vi "OPEN EXCEL.vi"(2 "错误输入（无错误）":errorcluster, 3 "Visible":bool, 4 "Excel._Application":refnum<k7>) -> (0 "错误输出":errorcluster, 1 "引用输出":refnum<k7>)   [LabVIEW 2018]
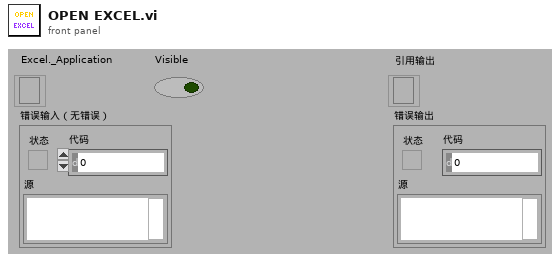
[diagram p1: front panel]
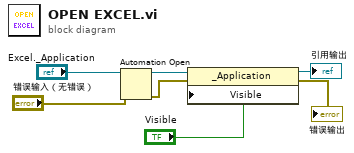
[diagram p0: block diagram]
diagram:
  n1 = Automation Open(error in (no error)="错误输入（无错误）", Automation Refnum="Excel._Application") -> (Automation Refnum=w5:refnum<k7>, error out=w4:errorcluster)  [unwired: 2 in]
  n2 = property class="_Application"(reference=w5, error in=w4, "Visible"="Visible") -> (reference out=→"引用输出":refnum<k7>, error out=→"错误输出":errorcluster)
